vi "Update-filter-vars.vi"(8 "error in":errorcluster, 11 "Data ref. in":refnum<data-value>) -> (0 "error IO":errorcluster, 3 "Data ref.":refnum<data-value>)   [LabVIEW 2013, in "CameraVision.lvlib" / "CV-Main.lvclass"]
uses:
  CV-Main.lvclass
  CV-Main.lvclass/CV-Main.ctl
  Configuration/CV-Configuration.lvclass/CV-Configuration.ctl
  Storage/CV-Storage.lvclass/CV-Storage.ctl
  Filter/CV-Filter.lvclass/CV-Filter.ctl
  UI/Module-states.ctl
  Storage/Read Storage directory.vi
  Storage/Read Storage prefix.vi
  Filter/Write Filter file labels.vi
  Filter/Write Filter file reference.vi
  Filter/Write Duration temp.vi
  Filter/Write Filter status.vi
  Read Filter params.vi
  Read Analysis params.vi
  Read Temperature params.vi
  Read Storage params.vi
  Read Config params.vi
  Configuration/Read Number of cameras.vi
  Storage/Read Layer index.vi
  Storage/Read Storage mode.vi
  Filter/Read Filter array temp.vi
  Filter/Read Filter file reference.vi
  Filter/CV-Filter.lvclass
  Analysis/CV-Analysis.lvclass
  Temperature/CV-Temperature.lvclass
  Storage/CV-Storage.lvclass
  Configuration/CV-Configuration.lvclass
  UI/CV-UI.lvclass
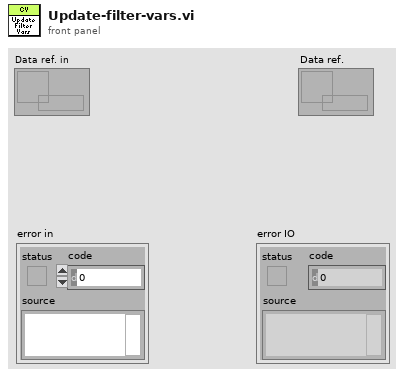
[diagram p1: front panel]
types:
  T1 = enum16{"1 file per layer", "1 file for all layers "}
  T2 = typedef "CameraVision.lvlib/CV-UI.lvclass/Module-states.ctl" = enum16{"Inactive", "Active", "Data-loss", "Error", "Simulation", "Synchronizing", "Initialized", "Released"}
  T3 = enum16{"open", "open or create", "create or replace", "create", "open (read-only)"}
  T4 = typedef "CameraVision.lvlib/CV-Filter.lvclass/Filter-characteristic.ctl" = enum16{"Average intensity [0-255]", "Peak intensity [0-255]", "Melt-pool size [mm²]", "Melt-pool aspect ratio []", "Melt-pool fragments []", "Melt-pool position X [pixel]", "Melt-pool position Y [pixel]", "Average temperature [°C]", "Max. temperature [°C]", "Min. temperature [°C]", "Std. dev. temperature [°C]"}
  T5 = typedef "CameraVision.lvlib/Filter.lvclass/Filter-settings.ctl" = cluster{"Characteristic":T6, "Monitor":bool, "Min.":dbl, "Max.":dbl, "Min. Thres.":dbl, "Min. Dur.":u16, "Report":bool}
  T6 = typedef "CameraVision.lvlib/Filter.lvclass/Filter-characteristic.ctl" = enum16{"Average intensity [0-255]", "Peak intensity [0-255]", "Melt-pool size [mm²]", "Melt-pool aspect ratio []", "Melt-pool fragments []", "Melt-pool position X [pixel]", "Melt-pool position Y [pixel]", "Average temperature [°C]", "Max. temperature [°C]", "Min. temperature [°C]", "Std. dev. temperature [°C]"}
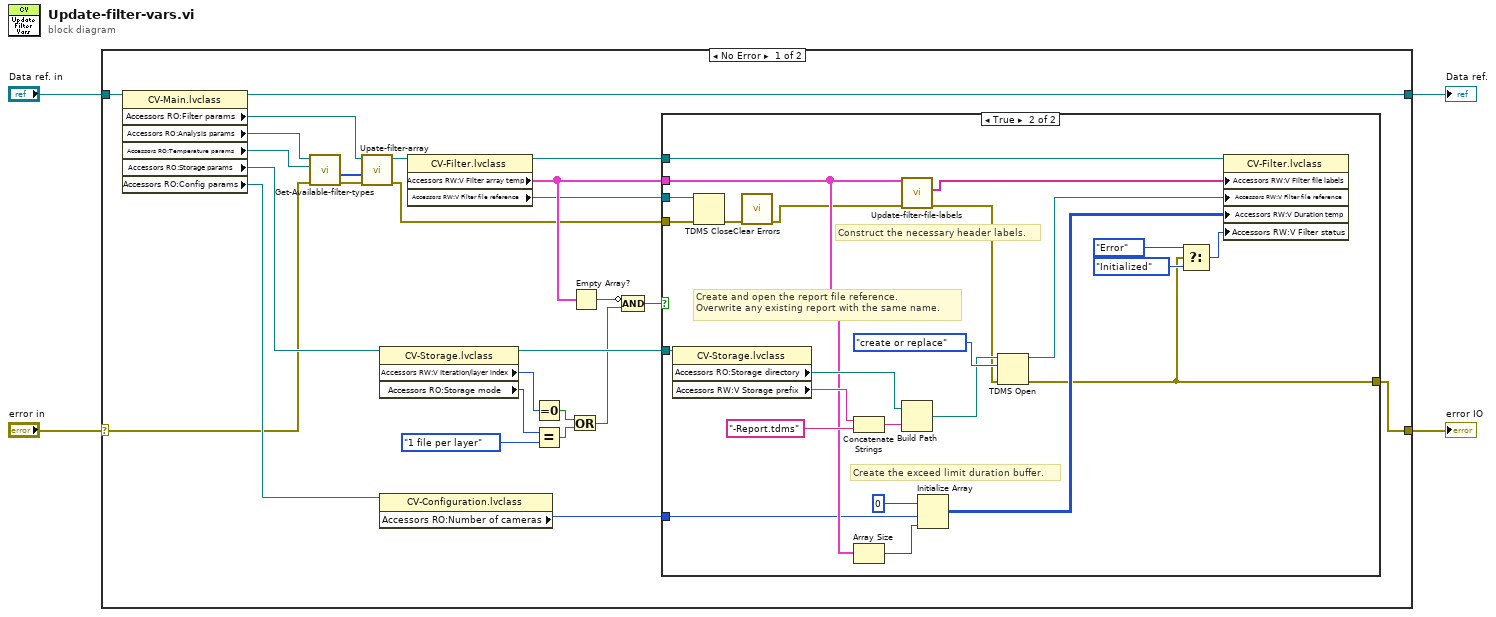
[diagram p0: block diagram]
diagram:
  n1 = case shown="No Error" "error in" {
    selector: "error in" -> [w6 w57]
    tunnel: [w12 w57] -> w3
    tunnel: "Data ref. in" -> [w29 w56]
    tunnel: [w11 w56] -> w1
    frame No Error {
      n2 = property class="CV-Main.lvclass"(reference=w29) -> (reference out=w11:refnum<data-value>, "Accessors RO:Filter params"=w10:refnum<data-value>, "Accessors RO:Analysis params"=w8:refnum<data-value>, "Accessors RO:Temperature params"=w7:refnum<data-value>, "Accessors RO:Storage params"=w28:refnum<data-value>, "Accessors RO:Config params"=w16:refnum<data-value>)  [unwired: 1 in, 1 out]
      n3 = call "Get-Available-filter-types.vi"("error in"=w6, "Temp. params. ref."=w7, "Analysis params. ref."=w8) -> ("error IO"=w5:errorcluster, "Available filters"=w9:T4[])  [unwired: 7 in]
      n4 = call "Upate-filter-array.vi"("error in"=w5, "Available filters"=w9, "Filter params. ref. in"=w10) -> ("error IO"=w13:errorcluster, "Filter params. ref."=w14:refnum<data-value>)  [unwired: 7 in]
      n5 = property class="CV-Storage.lvclass"(reference=w28) -> (reference out=w25:refnum<data-value>, "Accessors RW:V Iteration/layer index"=w21:u16, "Accessors RO:Storage mode"=w20:T1)  [unwired: 1 in, 1 out]
      n6 = property class="CV-Configuration.lvclass"(reference=w16) -> ("Accessors RO:Number of cameras"=w15:i32)  [unwired: 1 in, 2 out]
      n7 = property class="CV-Filter.lvclass"(reference=w14) -> (reference out=w30:refnum<data-value>, "Accessors RW:V Filter array temp"=w26:T5[], "Accessors RW:V Filter file reference"=w19:refnum<k34>)  [unwired: 1 in, 1 out]
      n8 = Equal To 0?(x=w21) -> (x = 0?=w23:bool)
      n9 = Equal?(x=w20, y=T1."1 file per layer") -> (x = y?=w22:bool)
      n10 = Or(x=w23, y=w22) -> (x .or. y?=w17:bool)
      n11 = Empty Array?(array=w26) -> (empty?=w27:bool)
      n12 = Compound Arithmetic op=AND(invert w27, w17) -> (w18:bool)
      n13 = case shown="True" w18 {
        tunnel: w30 -> [_ w55]
        tunnel: [w31 w32] -> w12
        tunnel: w26 -> [_ w46]
        tunnel: w25 -> [_ w42]
        tunnel: w19 -> [_ w41]
        tunnel: w15 -> [_ w39]
        tunnel: w13 -> [w31 w36]
        frame False {
        }
        frame True {
          # "Create the exceed limit duration buffer."
          # "Construct the necessary header labels."
          # "Create and open the report file reference.\nOverwrite any existing report with the same name."
          n14 = property class="CV-Storage.lvclass"(reference=w42) -> ("Accessors RO:Storage directory"=w51:path, "Accessors RW:V Storage prefix"=w50:string)  [unwired: 1 in, 2 out]
          n15 = TDMS Close(8:w36, 11:w41) -> (0:w40:errorcluster)  [unwired: 1 out]
          n16 = call <vilib>:"Clear Errors.vi"("error in (no error)"=w40) -> ("error out"=w37:errorcluster)  [unwired: 6 in]
          n17 = Concatenate Strings(w50, "-Report.tdms" ("string")) -> (w49:string)
          n18 = Array Size(array=w46) -> (size(s)=w44:i32)
          n19 = call "Update-filter-file-labels.vi"("error in"=w37, "Active filter array in"=w46) -> ("error IO"=w38:errorcluster, "Report labels"=w47:string[])  [unwired: 8 in]
          n20 = Build Path(base path=w51, name or relative path=w49) -> (appended path=w52:path)
          n21 = Initialize Array(u16 0, w39, w44) -> (w43:u16[][])
          n22 = TDMS Open(8:w38, 10:T3."create or replace" ("operation (0:open)"), 11:w52) -> (0:w32:errorcluster, 3:w48:refnum<k34>)  [unwired: 4 in]
          n23 = Select(t=Module-states."Error" ("Acquisition status"), s=w32, f=Module-states."Initialized" ("Acquisition status")) -> (s? t:f=w33:T2)
          n24 = property class="CV-Filter.lvclass"(reference=w55, "Accessors RW:V Filter file labels"=w47, "Accessors RW:V Filter file reference"=w48, "Accessors RW:V Duration temp"=w43, "Accessors RW:V Filter status"=w33) -> ()  [unwired: 1 in, 2 out]
        }
      }
    }
    frame Error {
    }
  }
  "error IO" <- w3
  "Data ref." <- w1
